vi "Set Ping.vi"(8 "error in (no error)":errorcluster, 9 "Ping Duration":dbl, 10 "Actor's Self Q":refnum<class "Message Enqueuer.lvclass">, 11 "Monitor Data in":refnum<class "Monitor Data.lvclass">) -> (0 "error out":errorcluster, 3 "Monitor Data out":refnum<class "Monitor Data.lvclass">)   [LabVIEW 2017, in "MGI-Monitored Actor Core.lvlib" / "Monitor Data.lvclass"]
doc: "Updates the ping duration for the actor\n\nCopyright: MGI 2016\nAuthor: Derek Trepanier"
uses:
  Monitor Data.lvclass
  <vilib>/ActorFramework/Message Enqueuer/Message Enqueuer.lvclass
  Monitor Data.lvclass/Monitor Data.ctl
  Actor Data.ctl
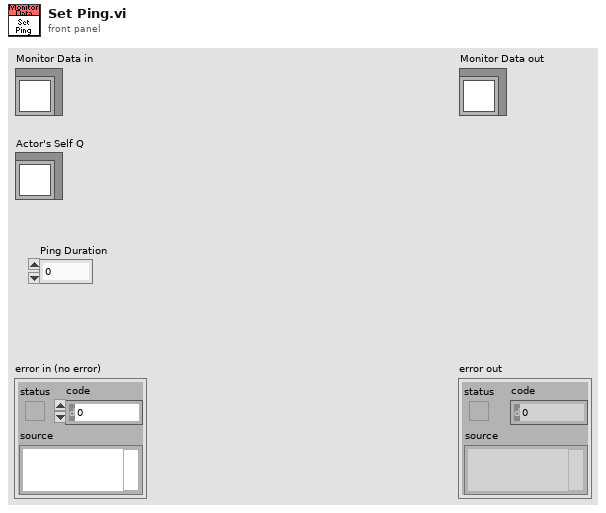
[diagram p1: front panel]
types:
  T1 = typedef "MGI-Monitored Actor Core.lvlib/Monitor Data.lvclass/Actor Data.ctl" = cluster{"Actor Type":string, "Actor Cores":string[], "Self":refnum<class "Message Enqueuer.lvclass">, "Caller":refnum<class "Message Enqueuer.lvclass">, "Actor Label":string, "Last Ping":dbl}
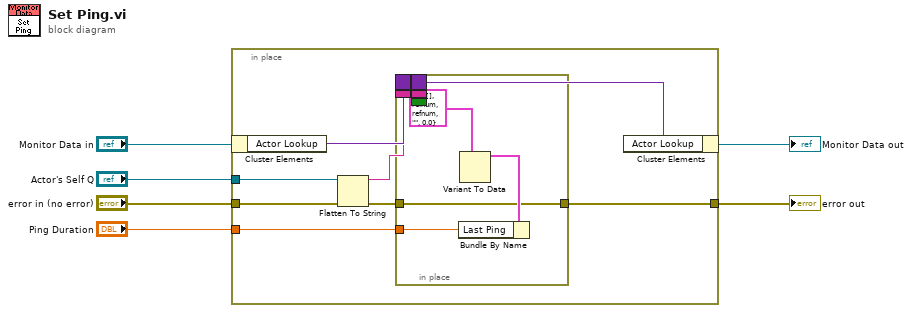
[diagram p0: block diagram]
diagram:
  n1 = in-place {
    in-place-border: "Actor's Self Q" -> [w14]
    in-place-border: "Ping Duration" -> [w13]
    in-place-border: "error in (no error)" -> [w12]
    in-place-border: [w8] -> w4
    n2 = in-place-cluster #1("Monitor Data in") -> ("Actor Lookup"=w11:variant)
    n3 = Flatten To String(anything=w14, error in (no error)=w12) -> (data string=w10:string, error out=w9:errorcluster)  [unwired: 2 in, 1 out]
    n4 = in-place {
      in-place-border: w13 -> [w20]
      border: w11 -> [_]
      border: w10 -> [_]
      border: [_] -> w7
      border: _ -> [_]
      border: _ -> [_]
      in-place-border: w9 -> [w15]
      in-place-border: [w15] -> w8
      n5 = Variant To Data(type=T1 {"Actor Type"="", "Actor Cores"=[], "Self"=refnum, "Caller"=refnum, "Actor Label"="", "Last Ping"=0.0} ("Actor Data"), Variant=w19) -> (data=w17:T1)  [unwired: 1 in, 1 out]
      n6 = Bundle By Name(cluster=w17, "Last Ping"=w20) -> (w16:T1)
    }
    n7 = in-place-cluster #1("Actor Lookup"=w7) -> (→"Monitor Data out":refnum<class "Monitor Data.lvclass">)
  }
  "error out" <- w4
